vi "Convert_to_2009_CORE.vi"(5 "TypeID":string, 7 "Type":T2, 8 "error in (no error)":errorcluster, 9 "ShortcutInfoIn":T3[](array[typedef]), 10 "FileInfoIn":T1[](array[typedef]), 11 "IB_Source_File in":refnum<class "IB_Source_File.lvclass">) -> (0 "error out":errorcluster, 1 "ShortcutInfoOut":T3[](array[typedef]), 2 "FileInfoOut":T1[](array[typedef]))   [LabVIEW 2020, in "IB_Source_File.lvclass"]
uses:
  <vilib>/AppBuilder/IB_Classes/Source/File/IB_Source_File.lvclass
  <vilib>/AppBuilder/IB_Classes/Source/File/IB_Source_File.lvclass/IB_Source_File.ctl
  <resource>/Framework/Providers/Builds/Installer/CDK_sTypeDef_BuildTypes.ctl
  <resource>/Framework/Providers/Builds/Installer/CDK_sTypeDef_FileInfo.ctl
  <vilib>/AppBuilder/IB_Classes/Source/IB_Source.lvclass
  <vilib>/AppBuilder/IB_Classes/Shortcut/IB_Shortcut.lvclass
  <resource>/Framework/Providers/Builds/Installer/CDK_sTypeDef_ShortcutInfo.ctl
  <resource>/Framework/Providers/Builds/Installer/CDK_GLOBAL_LABELS.vi
  e:/builds/penguin/labview/branches/2020/dev/dist/vi.lib/AppBuilder/IB_Classes/Source/IB_Source.lvclass
  e:/builds/penguin/labview/branches/2020/dev/dist/vi.lib/AppBuilder/IB_Classes/Source/File/IB_Source_File.lvclass
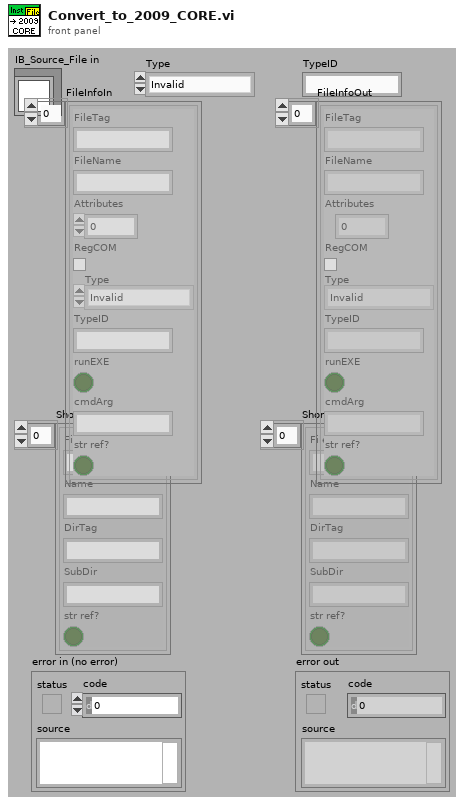
[diagram p1: front panel]
types:
  T1 = typedef "CDK_sTypeDef_FileInfo.ctl" = cluster{"FileTag":string, "FileName":string, "Attributes":i16, "RegCOM":bool, "Type":T2, "TypeID":string, "runEXE":bool, "cmdArg":string, "str ref?":bool}
  T2 = typedef "CDK_sTypeDef_BuildTypes.ctl" = enum16{"Invalid", "File", "Folder", "BuildRule", "Library"}
  T3 = typedef "CDK_sTypeDef_ShortcutInfo.ctl" = cluster{"FileTag":string, "Name":string, "DirTag":string, "SubDir":string, "str ref?":bool}
  T4 = typedef "IB_Source.ctl" = cluster{"name":string, "sourceTag":string, "destTag":string, "path":path, "eng_installPath":string, "UI_inBuild?":bool, "str ref?":bool}
  T5 = typedef "IB_Shortcut.ctl" = cluster{"name":string, "destIndex":i32, "subDir":string, "address":string}
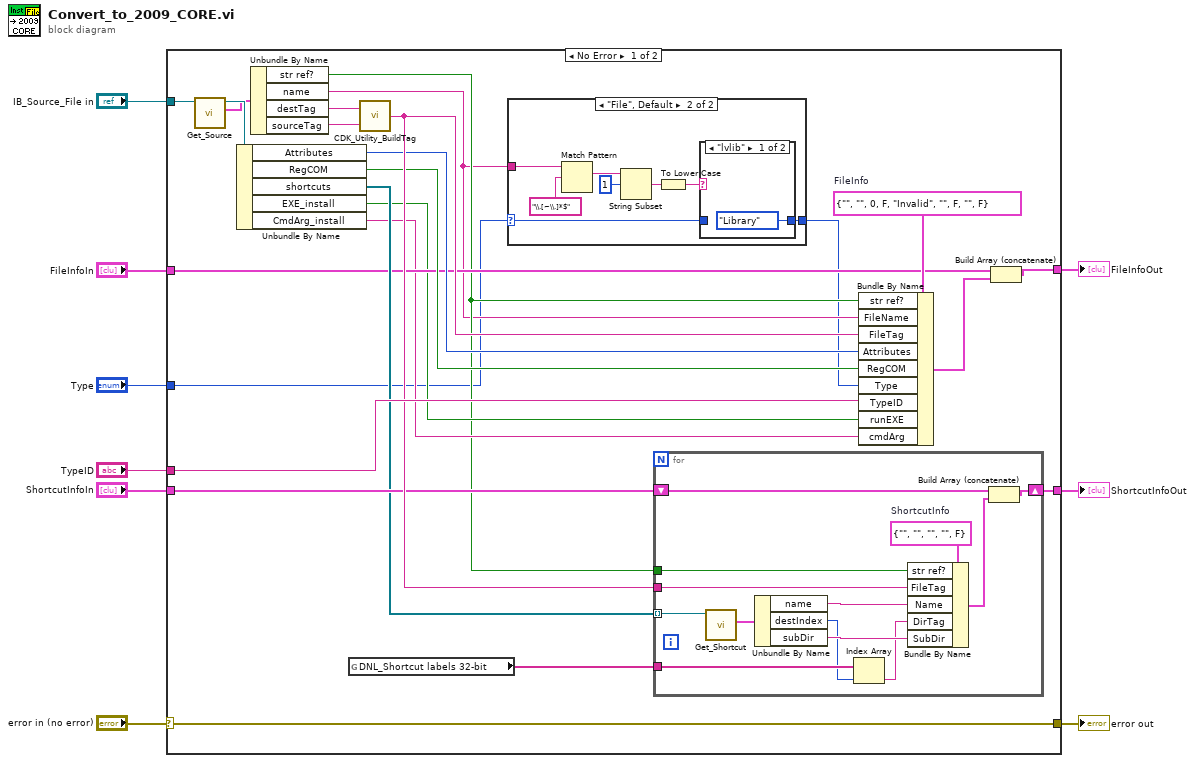
[diagram p0: block diagram]
diagram:
  n1 = case shown="No Error" "error in (no error)" {
    selector: "error in (no error)" -> [w18 w60]
    tunnel: "TypeID" -> [w33 _]
    tunnel: [w31 w58] -> w8
    tunnel: "ShortcutInfoIn" -> [w30 w58]
    tunnel: [w28 w59] -> w6
    tunnel: "Type" -> [w10 _]
    tunnel: "IB_Source_File in" -> [w22 _]
    tunnel: "FileInfoIn" -> [w19 w59]
    tunnel: [w18 w60] -> w1
    frame No Error {
      w20 = T1 {"FileTag"="", "FileName"="", "Attributes"=0, "RegCOM"=FALSE, "Type"=enum."Invalid", "TypeID"="", "runEXE"=FALSE, "cmdArg"="", "str ref?"=FALSE}  # FileInfo
      n2 = call <vilib>:"Get_Source.vi"("IB_Source in"=w22) -> ("data"=w23:T4, "IB_Source out"=w24:refnum<class "IB_Source_File.lvclass">)  [unwired: 1 in, 8 out]
      n3 = Unbundle By Name(w24) -> ("Attributes"=w25:i16, "RegCOM"=w26:bool, "shortcuts"=w29:refnum<class "IB_Shortcut.lvclass">[], "EXE_install"=w16:bool, "CmdArg_install"=w15:string)
      n4 = Unbundle By Name(w23) -> ("str ref?"=w13:bool, "name"=w12:string, "destTag"=w27:string, "sourceTag"=w17:string)
      n5 = global read "CDK_GLOBAL_LABELS.vi" "DNL_Shortcut labels 32-bit"() -> (w14:string[])
      n6 = call <resource>:"CDK_Utility_BuildTag.vi"("name or relative path"=w17, "BasePath"=w27) -> ("appended path"=w32:string)
      n7 = case shown="\"File\", Default" w10 {
        selector: w10 -> [w34 w35]
        tunnel: w12 -> [_ w38]
        tunnel: [w34 w37] -> w11
        frame "BuildRule" {
        }
        frame "File", Default {
          n8 = Match Pattern(string=w38, regular expression="\\.[~\\.]*$") -> (match substring=w42:string)  [unwired: 4 out]
          n9 = String Subset(string=w42, offset (0)=1) -> (substring=w41:string)  [unwired: 1 out]
          n10 = To Lower Case(string=w41) -> (all lower case string=w36:string)
          n11 = case shown="\"lvlib\"" w36 {
            tunnel: w35 -> [_ w44]
            tunnel: [CDK_sTypeDef_BuildTypes."Library" ("Type") w44] -> w37
            frame "lvlib" {
            }
            frame Default {
            }
          }
        }
      }
      n12 = for {
        tunnel: w29 -> [w57] mode=indexing
        shift-right: [w53] -> w31
        shift-left: w30 -> [w54]
        tunnel: w32 -> [w52]
        tunnel: w14 -> [w48]
        tunnel: w13 -> [w45]
        w49 = T3 {"FileTag"="", "Name"="", "DirTag"="", "SubDir"="", "str ref?"=FALSE}  # ShortcutInfo
        n13 = call <vilib>:"Get_Shortcut.vi"("Class in"=w57) -> ("data"=w55:T5)  [unwired: 1 in, 9 out]
        n14 = Unbundle By Name(w55) -> ("name"=w51:string, "destIndex"=w47:i32, "subDir"=w50:string)
        n15 = Index Array(array=w48, index=w47) -> (element=w46:string)
        n16 = Bundle By Name(cluster=w49, "str ref?"=w45, "FileTag"=w52, "Name"=w51, "DirTag"=w46, "SubDir"=w50) -> (w56:T3)
        n17 = Build Array (concatenate)(w54, w56) -> (w53:T3[])
      }
      n18 = Bundle By Name(cluster=w20, "str ref?"=w13, "FileName"=w12, "FileTag"=w32, "Attributes"=w25, "RegCOM"=w26, "Type"=w11, "TypeID"=w33, "runEXE"=w16, "cmdArg"=w15) -> (w21:T1)
      n19 = Build Array (concatenate)(w19, w21) -> (w28:T1[])
    }
    frame Error {
    }
  }
  "ShortcutInfoOut" <- w8
  "FileInfoOut" <- w6
  "error out" <- w1
